vi "Stop Core.vi"(10 "final error code":i32, 11 "Actor_UI_Template in":refnum<class "Actor_UI_Template.lvclass">) -> (3 "Actor_UI_Template out":refnum<class "Actor_UI_Template.lvclass">)   [LabVIEW 2020, in "Actor_UI_Template.lvlib" / "Actor_UI_Template.lvclass"]
doc: "(<B>Filename</B>: Actor Framework.lvlib:Actor.lvclass:Stop Core.vi)\n\nDefines what the actor does before it stops. Use the <B>final error code</B> input to determine whether the actor shut down in response to an error.\n\nBy default, this method passes the Stop message along to all auto-stop nested actors. A descendant class may override this method to define additional behavior, such as shutting down any processes the actor initiated in its override of the Actor Core method."
uses:
  Actor_UI_Template.lvclass
  Actor_UI_Template.lvclass/Actor_UI_Template.ctl
  <vilib>/ActorFramework/Actor/Actor.lvclass
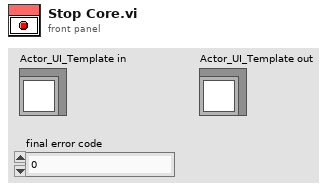
[diagram p1: front panel]
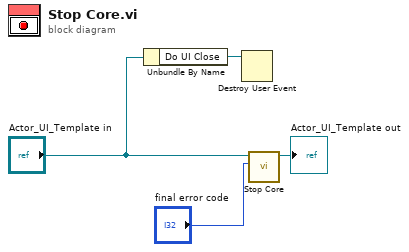
[diagram p0: block diagram]
diagram:
  n1 = Unbundle By Name("Actor_UI_Template in") -> ("Do UI Close"=w1:refnum<user-event>)
  n2 = Destroy User Event(user event=w1) -> ()  [unwired: 1 in, 1 out]
  n3 = call-parent "Stop Core.vi"("final error code"="final error code", "Actor in"="Actor_UI_Template in") -> ("Actor out"=→"Actor_UI_Template out":refnum<class "Actor_UI_Template.lvclass">)  [unwired: 9 in]
